vi "Init Ellipse.vi"(7 "Color (RGB black)":refnum<class "Color.lvclass">=refnum, 8 "error in (no error)":errorcluster, 9 "bottom right (0,0)":cluster{"x":i16, "y":i16}, 10 "top left (0,0)":cluster{"x":i16, "y":i16}, 11 "Ellipse in":refnum<class "Ellipse.lvclass">) -> (0 "error out":errorcluster, 3 "Ellipse out":refnum<class "Ellipse.lvclass">)   [LabVIEW 2018, in "Ellipse.lvclass"]
doc: "Initialize an ellipse"
uses:
  Ellipse.lvclass
  Color/Color.lvclass
  RGB Color/RGB Color.lvclass
  Ellipse.lvclass/Ellipse.ctl
  Graphics Object/Graphics Object.lvclass
panel:
  # "expressionflow.com"
  # "Copyright (c) 2008 Tomi Maila. All rights reserved."
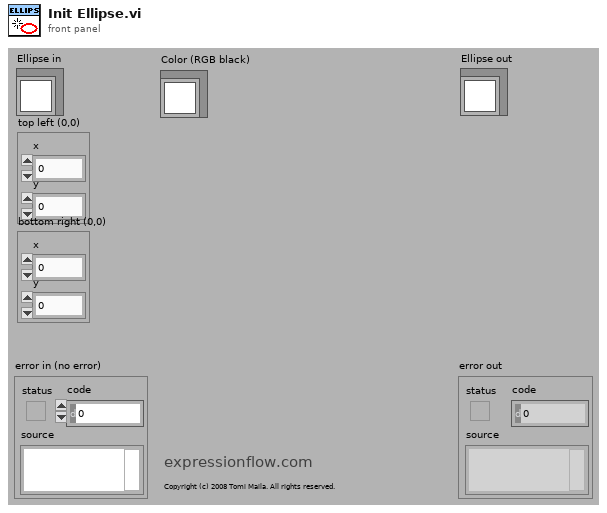
[diagram p1: front panel]
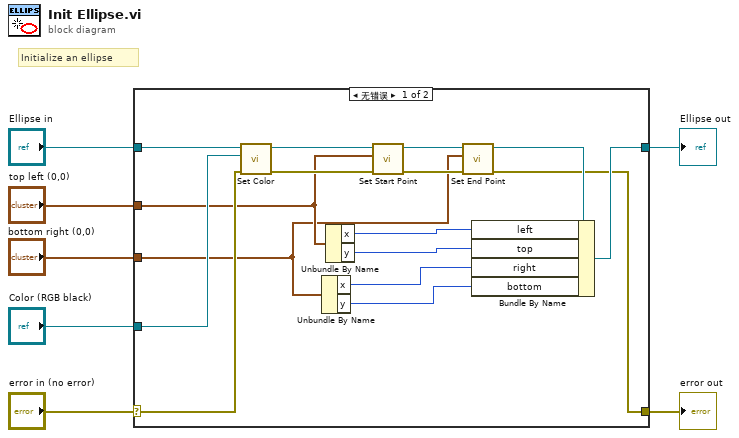
[diagram p0: block diagram]
diagram:
  # "Initialize an ellipse"
  n1 = case shown="无错误" "error in (no error)" {
    selector: "error in (no error)" -> [w21 w25]
    tunnel: [w8 w25] -> w6
    tunnel: [w23 w24] -> w4
    tunnel: "Ellipse in" -> [w22 w24]
    tunnel: "top left (0,0)" -> [w13 _]
    tunnel: "bottom right (0,0)" -> [w10 _]
    tunnel: "Color (RGB black)" -> [w20 _]
    frame No Error {
      n2 = call-dynamic "Set Color.vi"("error in (no error)"=w21, "Color (RGB black)"=w20, "Geometric Object.lvclass in"=w22) -> ("error out"=w14:errorcluster, "Geometric Object.lvclass out"=w15:refnum<class "Ellipse.lvclass">)  [unwired: 7 in]
      n3 = Unbundle By Name(w10) -> ("x"=w17:i16, "y"=w16:i16)
      n4 = Unbundle By Name(w13) -> ("x"=w19:i16, "y"=w18:i16)
      n5 = call "Set Start Point.vi"("error in (no error)"=w14, "start point (0,0)"=w13, "Graphics Object.lvclass in"=w15) -> ("error out"=w11:errorcluster, "Graphics Object.lvclass out"=w12:refnum<class "Ellipse.lvclass">)  [unwired: 7 in]
      n6 = call "Set End Point.vi"("error in (no error)"=w11, "end point (0,0)"=w10, "Graphics Object.lvclass in"=w12) -> ("error out"=w8:errorcluster, "Graphics Object.lvclass out"=w9:refnum<class "Ellipse.lvclass">)  [unwired: 7 in]
      n7 = Bundle By Name(cluster=w9, "left"=w19, "top"=w18, "right"=w17, "bottom"=w16) -> (w23:refnum<class "Ellipse.lvclass">)
    }
    frame Error {
    }
  }
  "error out" <- w6
  "Ellipse out" <- w4
